vi "AnnexDSim.vi"(8 "error in (no error)":errorcluster, 11 "C37.118 Sim in":refnum<class "C37.118 Sim.lvclass">) -> (0 "error out":errorcluster, 3 "C37.118 Sim out":refnum<class "C37.118 Sim.lvclass">)   [LabVIEW 2018, in "SensorPlugins.lvlib" / "C37.118 Sim.lvclass"]
uses:
  C37.118 Sim.lvclass
  C:/projects/ICDAS/NistPluggableModules/Sensor/SensorPlugins/PmuBaseClass/PmuBase.lvclass
  C37.118 Sim.lvclass/C37.118 Sim.ctl
  PmuBaseClass/PmuBase.lvclass/PmuBase.ctl
  PmuBaseClass/Typedef/PmuData.ctl
  Accessors/Read Function.vi
  PmuBaseClass/Accessors/Read PmuConfig.vi
  Accessors/Read Time.vi
  PmuBaseClass/Accessors/Write PmuDataArray.vi
  FGen/MemberClasses/FunctionBaseClass/FunctionBase.lvclass
  PmuBaseClass/PmuBase.lvclass
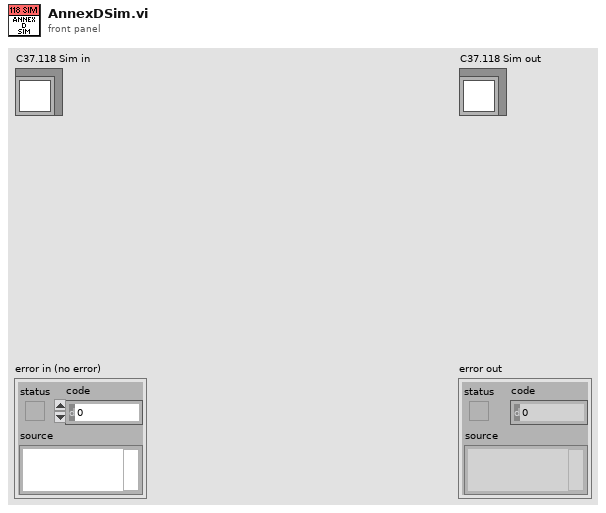
[diagram p1: front panel]
types:
  T1 = typedef "SensorPlugins.lvlib/PmuBase.lvclass/PmuData.ctl" = cluster{"Timestamp":dbl, "Synx":cdb[], "Freq":dbl, "ROCOF":dbl, "ID":i16}
  T2 = typedef "SensorPlugins.lvlib/PmuBase.lvclass/PmuConfig.ctl" = cluster{"Class":enum16{"M", "P"}, "Fs":i32, "F0":i32, "FSamp":i32, "SettlingTime":dbl, "T0":ext}
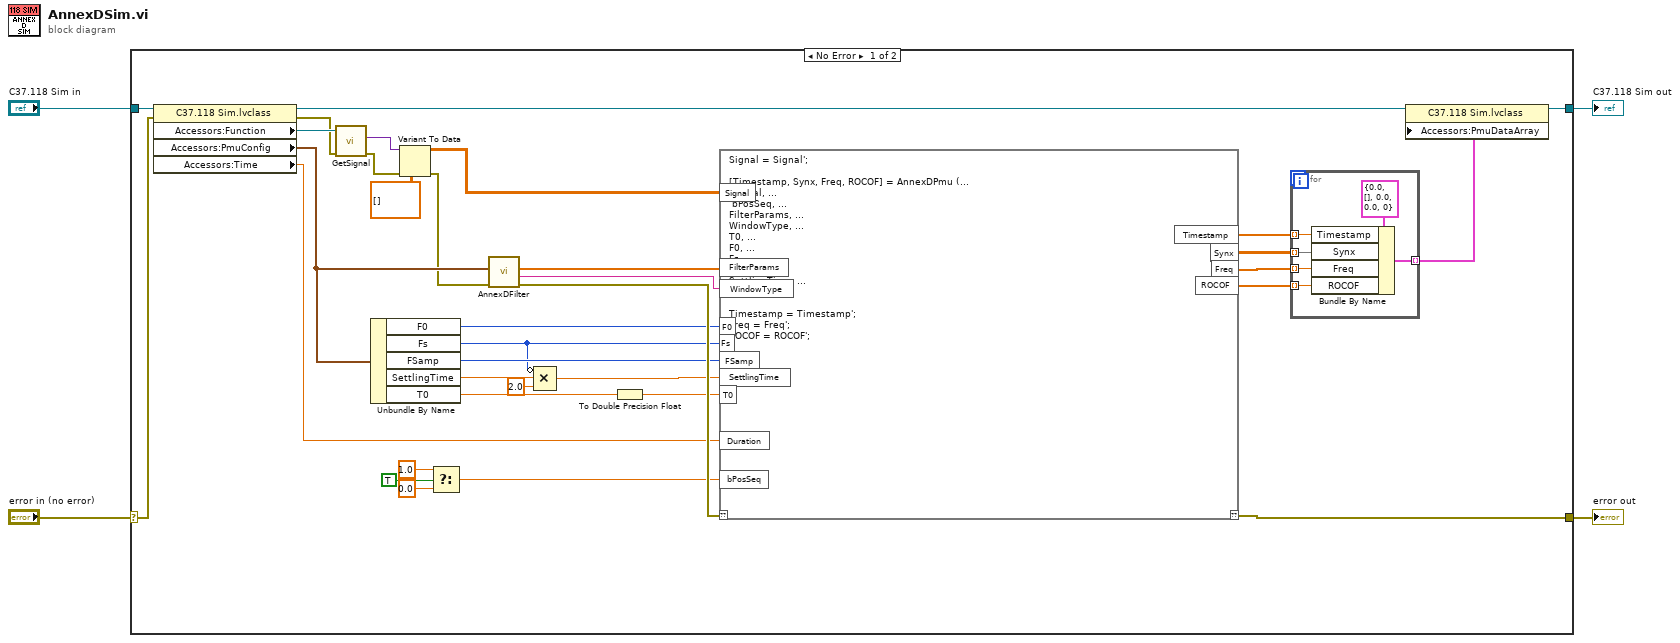
[diagram p0: block diagram]
diagram:
  n1 = case shown="No Error" "error in (no error)" {
    selector: "error in (no error)" -> [w36 w46]
    tunnel: [w28 w46] -> w3
    tunnel: [w23 w45] -> w1
    tunnel: "C37.118 Sim in" -> [w37 w45]
    frame No Error {
      n2 = property class="C37.118 Sim.lvclass"(reference=w37, error in=w36) -> (reference out=w38:refnum<class "C37.118 Sim.lvclass">, error out=w11:errorcluster, "Accessors:Function"=w12:refnum<class "FunctionBase.lvclass">, "Accessors:PmuConfig"=w35:T2, "Accessors:Time"=w5:ext)
      n3 = call-dynamic "GetSignal.vi"("error in (no error)"=w11, "FunctionBase in"=w12) -> ("error out"=w7:errorcluster, "Signal"=w10:variant)  [unwired: 7 in, 1 out]
      n4 = Unbundle By Name(w35) -> ("F0"=w30:i32, "Fs"=w20:i32, "FSamp"=w29:i32, "SettlingTime"=w19:dbl, "T0"=w21:ext)
      n5 = Variant To Data(error in=w7, type=dbl[][] [], Variant=w10) -> (data=w8:dbl[][], error out=w6:errorcluster)
      n6 = Select(t=1.0, s=TRUE, f=0.0) -> (s? t:f=w14:dbl)
      n7 = call "AnnexDFilter.vi"("error in (no error)"=w6, "PmuConfig"=w35) -> ("error out"=w32:errorcluster, "WindowType"=w33:string, "FilterParams"=w34:dbl[])  [unwired: 7 in]
      n8 = Compound Arithmetic op=MULTIPLY(invert w20, w19, 2.0 ("value")) -> (w17:dbl)
      n9 = To Double Precision Float(number=w21) -> (double precision float=w13:dbl)
      n10 = script code="Signal = Signal';\n\n[Timestamp, Synx, Freq, ROCOF] = AnnexDPmu (...\n Signal, ...\n bPosSeq, ...\nFilterParams, ...\nWindowType, ...\nT0, ...\nF0, ...\nFs, ...\nFSamp, ...\nSettlingTime, ...\nDuration);\n\nTimestamp = Timestamp';\nFreq = Freq';\nROCOF = ROCOF';"("??"=w32, "Signal"=w8, "bPosSeq"=w14, "FilterParams"=w34, "WindowType"=w33, "F0"=w30, "Fs"=w20, "FSamp"=w29, "SettlingTime"=w17, "T0"=w13, "Duration"=w5) -> ("??"=w28:errorcluster, "Timestamp"=w27:dbl[], "Synx"=w24:cdb[][], "Freq"=w26:dbl[], "ROCOF"=w25:dbl[])
      n11 = for {
        tunnel: w27 -> [w44] mode=indexing
        tunnel: w26 -> [w42] mode=indexing
        tunnel: w25 -> [w41] mode=indexing
        tunnel: w24 -> [w43] mode=indexing
        tunnel: [w40] -> w22 mode=indexing
        n12 = Bundle By Name(cluster=T1 {"Timestamp"=0.0, "Synx"=[], "Freq"=0.0, "ROCOF"=0.0, "ID"=0} ("PmuReport"), "Timestamp"=w44, "Synx"=w43, "Freq"=w42, "ROCOF"=w41) -> (w40:T1)
      }
      n13 = property class="C37.118 Sim.lvclass"(reference=w38, "Accessors:PmuDataArray"=w22) -> (reference out=w23:refnum<class "C37.118 Sim.lvclass">)  [unwired: 1 in, 1 out]
    }
    frame Error {
    }
  }
  "error out" <- w3
  "C37.118 Sim out" <- w1
